vi "Write Report.vi"(8 "error in (no error)":errorcluster, 10 "Resource In":variant, 11 "Analyze Results SHG-AK in":refnum<class "Analyze Results SHG-AK.lvclass">) -> (0 "error out":errorcluster, 2 "Resource Out":variant, 3 "Analyze Results SHG-AK out":refnum<class "Analyze Results SHG-AK.lvclass">)   [LabVIEW 2014, in "Analyze Results SHG-AK.lvclass"]
uses:
  Analyze Results SHG-AK.lvclass
  <vilib>/Utility/config.llb/Config Data RefNum.ctl
  Analyze Results SHG-AK.lvclass/Analyze Results SHG-AK.ctl
  Results Base/Analyze Results Base.lvclass/Analyze Results Base.ctl
  Results Base/Read Section.vi
  <vilib>/Utility/config.llb/Write Key (Double).vi
  <vilib>/Utility/config.llb/NI_LVConfig.lvlib
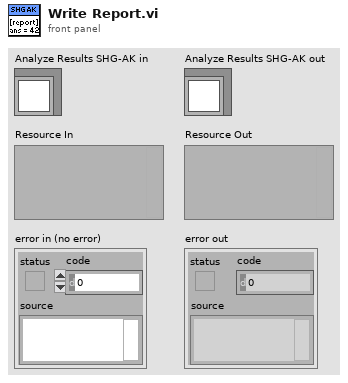
[diagram p1: front panel]
types:
  T1 = typedef "NI_LVConfig.lvlib/Config Data RefNum.ctl" = refnum<k1>
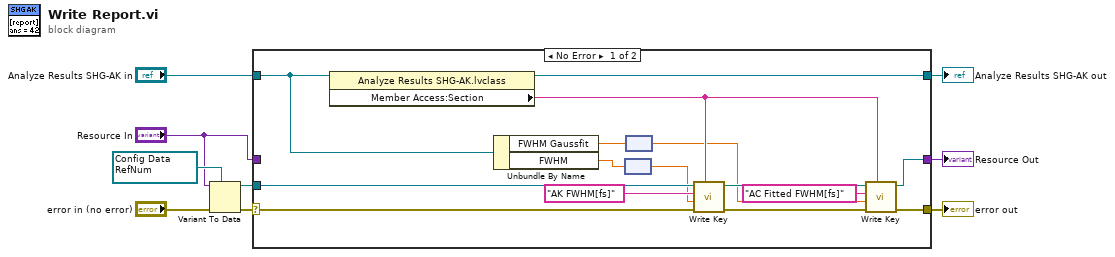
[diagram p0: block diagram]
diagram:
  w9 = T1 refnum items=["config data"] ("refnum")
  n1 = Variant To Data(error in="error in (no error)", type=w9, Variant="Resource In") -> (data=w8:T1, error out=w7:errorcluster)
  n2 = case shown="No Error" w7 {
    selector: w7 -> [w21 w26]
    tunnel: w8 -> [w22 _]
    tunnel: "Analyze Results SHG-AK in" -> [w10 w25]
    tunnel: [w24 w25] -> w3
    tunnel: [w19 w27] -> w2
    tunnel: [w18 w26] -> w1
    tunnel: "Resource In" -> [_ w27]
    frame No Error {
      n3 = property class="Analyze Results SHG-AK.lvclass"(reference=w10) -> (reference out=w24:refnum<class "Analyze Results SHG-AK.lvclass">, "Member Access:Section"=w20:string)  [unwired: 1 in, 1 out]
      n4 = Unbundle By Name(w10) -> ("FWHM Gaussfit"=w15:dbl[unit], "FWHM"=w12:dbl[unit])
      n5 = node(w12) -> (w11:dbl)
      n6 = node(w15) -> (w14:dbl)
      n7 = call-poly <vilib>:"Write Key.vi"("section"=w20, "error in (no error)"=w21, "value"=w11, "key"="AK FWHM[fs]", "refnum"=w22) -> ("error out"=w17:errorcluster, "refnum out"=w23:T1)  [unwired: 4 in, 1 out]
      n8 = call-poly <vilib>:"Write Key.vi"("section"=w20, "error in (no error)"=w17, "value"=w14, "key"="AC Fitted FWHM[fs]", "refnum"=w23) -> ("error out"=w18:errorcluster, "refnum out"=w19:T1)  [unwired: 4 in, 1 out]
    }
    frame Error {
    }
  }
  "error out" <- w1
  "Analyze Results SHG-AK out" <- w3
  "Resource Out" <- w2
